vi "Add Step to Tree.vi"(9 "Step Index":i32, 10 "Step Settings":T1, 11 "UI Data In":refnum<class "Settings UI.lvclass">) -> (1 "Tree Items":T2(array[cluster]), 2 "Step tag":string, 3 "UI Data out":refnum<class "Settings UI.lvclass">)   [LabVIEW 2020, in "Output Sequencer.lvlib" / "Settings UI.lvclass"]
uses:
  Settings UI.lvclass
  Types/Step Settings.ctl
  Types/Tree Index Enum.ctl
  Globals/Global Tree Data.vi
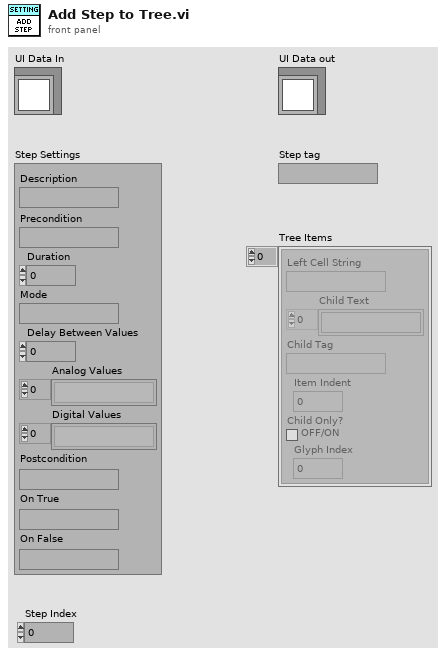
[diagram p1: front panel]
types:
  T1 = typedef "Output Sequencer.lvlib/Settings UI.lvclass/Step Settings.ctl" = cluster{"Description":string, "Precondition":string, "Duration":dbl, "Mode":string, "Delay Between Values":dbl, "Analog Values":string[], "Digital Values":string[], "Postcondition":string, "On True":string, "On False":string}
  T2 = cluster{"Left Cell String":string, "Child Text":string[], "Child Tag":string, "Item Indent":i32, "Child Only?":bool, "Glyph Index":i32}[]
  T3 = typedef "Output Sequencer.lvlib/Settings UI.lvclass/Tree Index Enum.ctl" = enum16{"General Settings", "Num Steps", "Num Analog", "Num Digital", "Show Confirmation", "Interp Priority", "Adv Timing", "Enable Conditions", "Seq Execution", "Reset Test Start", "Only When Test", "Delay After Test", "Start condition", "Re-triggering", "Stop condition", "Stop After Cycles", "Stop Values", "Default Values", "Default Analog", "Default Digital", "Steps", "Step #", "Description", "Precondition", "Duration", "Mode", "Delay Between Vals", "Analog Values", "Digital Values", "Postcondition", "On True", "On False"}
  T4 = cluster{"Left Cell String":string, "Child Text":string[], "Child Tag":string, "Item Indent":i32, "Child Only?":bool, "Glyph Index":i32}
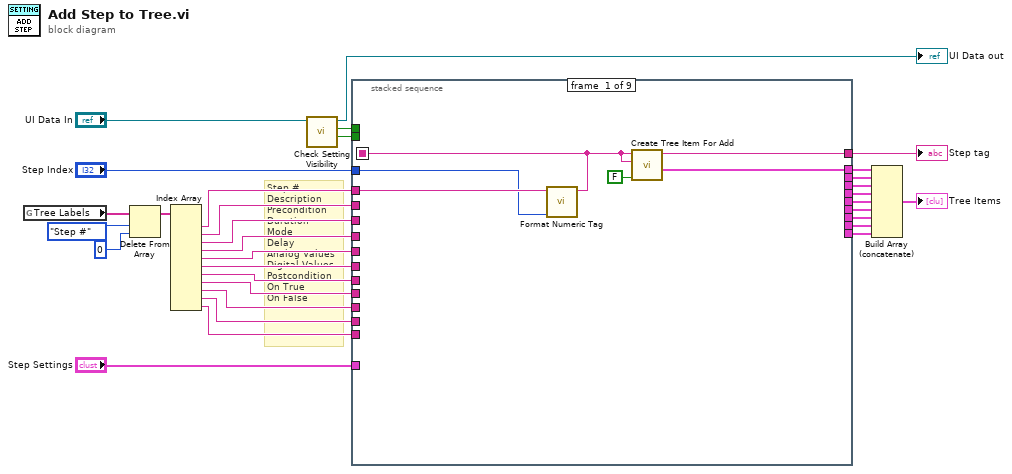
[diagram p0: block diagram]
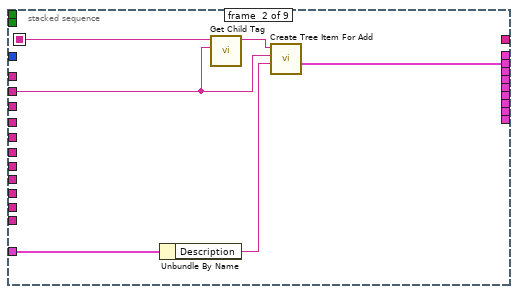
[diagram p2: hidden frame]
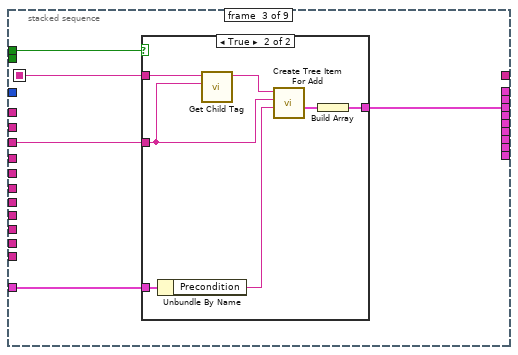
[diagram p3: hidden frame]
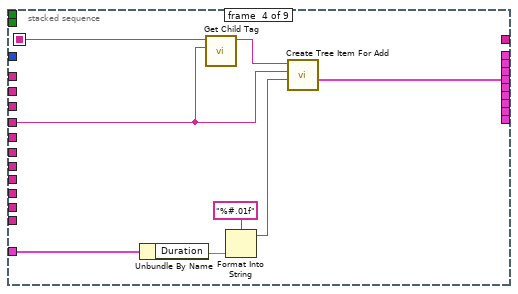
[diagram p5: hidden frame]
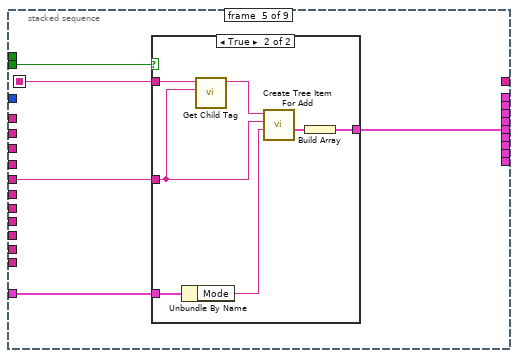
[diagram p6: hidden frame]
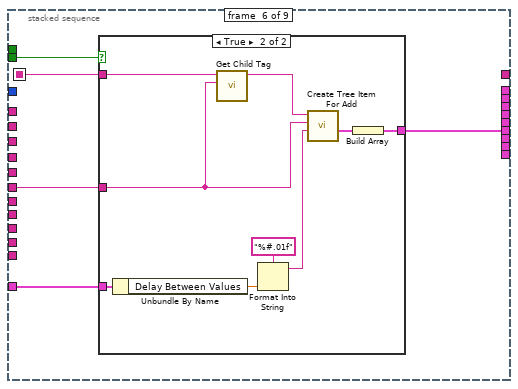
[diagram p8: hidden frame]
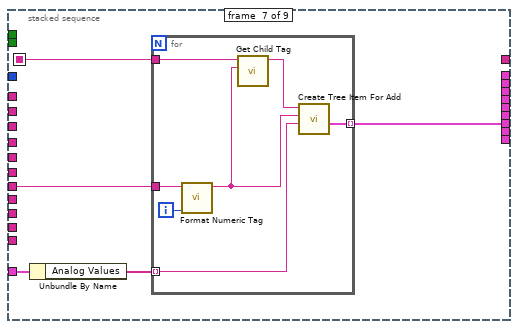
[diagram p10: hidden frame]
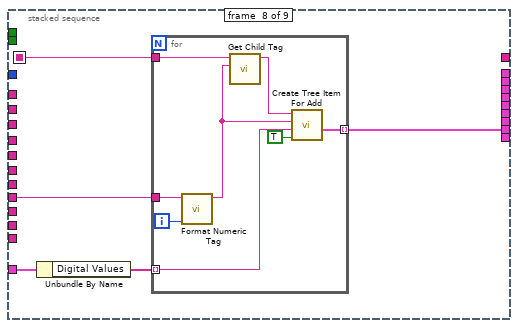
[diagram p11: hidden frame]
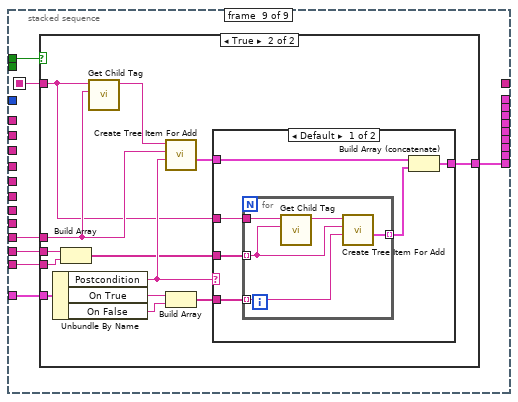
[diagram p12: hidden frame]
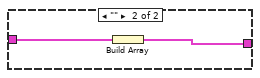
[diagram p14: hidden frame]
diagram:
  # "Step #\nDescription\nPrecondition\nDuration\nMode\nDelay\nAnalog Values\nDigital Values\nPostcondition\nOn True\nOn False"
  n1 = global read "Global Tree Data.vi" "Tree Labels"() -> (w14:string[])
  n2 = Delete From Array(array=w14, length=Tree_Index_Enum."Step #" ("Tree Index Enum"), index=0) -> (array with subset deleted=w21:string[])  [unwired: 1 out]
  n3 = Index Array(array=w21) -> (element #1=w20:string, element #2=w16:string, element #3=w17:string, element #4=w18:string, element #5=w19:string, element #6=w15:string, element #7=w13:string, element #8=w11:string, element #9=w9:string, element #10=w8:string, element #11=w7:string)  [unwired: 11 in]
  n4 = call "Check Setting Visibility.vi"("UI Data in"="UI Data In") -> ("Advanced timing visible"=w3:bool, "Conditional settings visible"=w2:bool, "UI Data out"=→"UI Data out":refnum<class "Settings UI.lvclass">)  [unwired: 7 in, 1 out]
  n5 = stacked-sequence {
    seq-local: [w33 _ _ _ _ _ _ _ _] -> [_ w41 w49 w59 w69 w81 w95 w107 w119]
    tunnel: "Step Index" -> [w34 _ _ _ _ _ _ _ _]
    tunnel: w20 -> [w35 _ _ _ _ _ _ _ _]
    tunnel: [w37 _ _ _ _ _ _ _ _] -> w29
    tunnel: w16 -> [_ w40 _ _ _ _ _ _ _]
    tunnel: [w38 _ _ _ _ _ _ _ _] -> w23
    tunnel: [_ _ w47 _ _ _ _ _ _] -> w24
    tunnel: "Step Settings" -> [_ w44 w48 w64 w68 w80 w92 w104 w122]
    tunnel: w17 -> [_ _ w46 _ _ _ _ _ _]
    tunnel: [_ _ _ w60 _ _ _ _ _] -> w25
    tunnel: w18 -> [_ _ _ w58 _ _ _ _ _]
    tunnel: w3 -> [_ _ _ _ w67 w79 _ _ _]
    tunnel: [_ _ _ _ w65 _ _ _ _] -> w26
    tunnel: w19 -> [_ _ _ _ w66 _ _ _ _]
    tunnel: [_ _ _ _ _ w77 _ _ _] -> w27
    tunnel: [_ _ _ _ _ _ w93 _ _] -> w28
    tunnel: w15 -> [_ _ _ _ _ w78 _ _ _]
    tunnel: w13 -> [_ _ _ _ _ _ w94 _ _]
    tunnel: [_ w43 _ _ _ _ _ _ _] -> w12
    tunnel: w11 -> [_ _ _ _ _ _ _ w106 _]
    tunnel: [_ _ _ _ _ _ _ w105 _] -> w10
    tunnel: w9 -> [_ _ _ _ _ _ _ _ w121]
    tunnel: w8 -> [_ _ _ _ _ _ _ _ w118]
    tunnel: w7 -> [_ _ _ _ _ _ _ _ w117]
    tunnel: [_ _ _ _ _ _ _ _ w120] -> w6
    tunnel: w2 -> [_ _ w45 _ _ _ _ _ w116]
    frame #0 {
      n6 = call "Format Numeric Tag.vi"("Number"=w34, "Tree label"=w35) -> ("Tag"=w33:string)  [unwired: 9 in]
      n7 = call "Create Tree Item For Add.vi"("Child Only? (true)"=FALSE ("Child Only?"), "Left Cell String"=w33, "Child Tag in"=w33) -> ("Item"=w38:T4, "Child Tag out"=w37:string)  [unwired: 7 in]
    }
    frame #1 {
      n8 = Unbundle By Name(w44) -> ("Description"=w42:string)
      n9 = call "Get Child Tag.vi"("Child label"=w40, "Parent tag"=w41) -> ("Child tag"=w39:string)  [unwired: 9 in]
      n10 = call "Create Tree Item For Add.vi"("Child Text"=w42, "Left Cell String"=w40, "Child Tag in"=w39) -> ("Item"=w43:T4)  [unwired: 7 in, 1 out]
    }
    frame #2 {
      n11 = case shown="True" w45 {
        tunnel: w49 -> [_ w52]
        tunnel: w48 -> [_ w56]
        tunnel: [_ w54] -> w47
        tunnel: w46 -> [_ w51]
        frame False {
        }
        frame True {
          n12 = Unbundle By Name(w56) -> ("Precondition"=w55:string)
          n13 = call "Get Child Tag.vi"("Child label"=w51, "Parent tag"=w52) -> ("Child tag"=w50:string)  [unwired: 9 in]
          n14 = call "Create Tree Item For Add.vi"("Child Text"=w55, "Left Cell String"=w51, "Child Tag in"=w50) -> ("Item"=w53:T4)  [unwired: 7 in, 1 out]
          n15 = Build Array(w53) -> (w54:T2)
        }
      }
    }
    frame #3 {
      n16 = Unbundle By Name(w64) -> ("Duration"=w63:dbl)
      n17 = call "Get Child Tag.vi"("Child label"=w58, "Parent tag"=w59) -> ("Child tag"=w57:string)  [unwired: 9 in]
      n18 = Format Into String(format string="%#.01f", w63) -> (resulting string=w61:string)  [unwired: 2 in, 1 out]
      n19 = call "Create Tree Item For Add.vi"("Child Text"=w61, "Left Cell String"=w58, "Child Tag in"=w57) -> ("Item"=w60:T4)  [unwired: 7 in, 1 out]
    }
    frame #4 {
      n20 = case shown="True" w67 {
        tunnel: w69 -> [_ w71]
        tunnel: w68 -> [_ w76]
        tunnel: w66 -> [_ w72]
        tunnel: [_ w74] -> w65
        frame False {
        }
        frame True {
          n21 = Unbundle By Name(w76) -> ("Mode"=w73:string)
          n22 = call "Get Child Tag.vi"("Child label"=w72, "Parent tag"=w71) -> ("Child tag"=w70:string)  [unwired: 9 in]
          n23 = call "Create Tree Item For Add.vi"("Child Text"=w73, "Left Cell String"=w72, "Child Tag in"=w70) -> ("Item"=w75:T4)  [unwired: 7 in, 1 out]
          n24 = Build Array(w75) -> (w74:T2)
        }
      }
    }
    frame #5 {
      n25 = case shown="True" w79 {
        tunnel: w81 -> [_ w83]
        tunnel: w80 -> [_ w90]
        tunnel: [_ w88] -> w77
        tunnel: w78 -> [_ w84]
        frame False {
          # "If no analog or digital channels configured, no need for delay since this only applies to channels."
        }
        frame True {
          n26 = Unbundle By Name(w90) -> ("Delay Between Values"=w86:dbl)
          n27 = call "Get Child Tag.vi"("Child label"=w84, "Parent tag"=w83) -> ("Child tag"=w82:string)  [unwired: 9 in]
          n28 = Format Into String(format string="%#.01f", w86) -> (resulting string=w85:string)  [unwired: 2 in, 1 out]
          n29 = call "Create Tree Item For Add.vi"("Child Text"=w85, "Left Cell String"=w84, "Child Tag in"=w82) -> ("Item"=w89:T4)  [unwired: 7 in, 1 out]
          n30 = Build Array(w89) -> (w88:T2)
        }
      }
    }
    frame #6 {
      n31 = Unbundle By Name(w92) -> ("Analog Values"=w91:string[])
      n32 = for {
        tunnel: w95 -> [w100]
        tunnel: w94 -> [w98]
        tunnel: [w102] -> w93 mode=indexing
        tunnel: w91 -> [w101] mode=indexing
        i -> [w97]
        n33 = call "Format Numeric Tag.vi"("Number"=w97, "Tree label"=w98) -> ("Tag"=w96:string)  [unwired: 9 in]
        n34 = call "Get Child Tag.vi"("Child label"=w96, "Parent tag"=w100) -> ("Child tag"=w99:string)  [unwired: 9 in]
        n35 = call "Create Tree Item For Add.vi"("Child Text"=w101, "Left Cell String"=w96, "Child Tag in"=w99) -> ("Item"=w102:T4)  [unwired: 7 in, 1 out]
      }
    }
    frame #7 {
      n36 = Unbundle By Name(w104) -> ("Digital Values"=w103:string[])
      n37 = for {
        tunnel: w107 -> [w112]
        tunnel: w106 -> [w110]
        tunnel: [w115] -> w105 mode=indexing
        tunnel: w103 -> [w114] mode=indexing
        i -> [w109]
        n38 = call "Format Numeric Tag.vi"("Number"=w109, "Tree label"=w110) -> ("Tag"=w108:string)  [unwired: 9 in]
        n39 = call "Get Child Tag.vi"("Child label"=w108, "Parent tag"=w112) -> ("Child tag"=w111:string)  [unwired: 9 in]
        n40 = call "Create Tree Item For Add.vi"("Child Only? (true)"=TRUE ("Child Only?"), "Child Text"=w114, "Left Cell String"=w108, "Child Tag in"=w111) -> ("Item"=w115:T4)  [unwired: 6 in, 1 out]
      }
    }
    frame #8 {
      n41 = case shown="True" w116 {
        tunnel: w122 -> [_ w135]
        tunnel: w121 -> [_ w125]
        tunnel: [_ w132] -> w120
        tunnel: w119 -> [_ w124]
        tunnel: w118 -> [_ w131]
        tunnel: w117 -> [_ w130]
        frame False {
        }
        frame True {
          n42 = Unbundle By Name(w135) -> ("Postcondition"=w134:string, "On True"=w129:string, "On False"=w128:string)
          n43 = Build Array(w131, w130) -> (w126:string[])
          n44 = call "Get Child Tag.vi"("Child label"=w125, "Parent tag"=w124) -> ("Child tag"=w123:string)  [unwired: 9 in]
          n45 = call "Create Tree Item For Add.vi"("Child Text"=w134, "Left Cell String"=w125, "Child Tag in"=w123) -> ("Item"=w133:T4)  [unwired: 7 in, 1 out]
          n46 = Build Array(w129, w128) -> (w127:string[])
          n47 = case shown="Default" w134 {
            tunnel: w133 -> [w138 w148]
            tunnel: [w137 w147] -> w132
            tunnel: w124 -> [w141 _]
            tunnel: w127 -> [w140 _]
            tunnel: w126 -> [w139 _]
            frame Default {
              n48 = for {
                tunnel: w141 -> [w144]
                tunnel: w140 -> [w146] mode=indexing
                tunnel: w139 -> [w143] mode=indexing
                tunnel: [w145] -> w136 mode=indexing
                n49 = call "Get Child Tag.vi"("Child label"=w143, "Parent tag"=w144) -> ("Child tag"=w142:string)  [unwired: 9 in]
                n50 = call "Create Tree Item For Add.vi"("Child Text"=w146, "Left Cell String"=w143, "Child Tag in"=w142) -> ("Item"=w145:T4)  [unwired: 7 in, 1 out]
              }
              n51 = Build Array (concatenate)(w138, w136) -> (w137:T2)
            }
            frame "" {
              n52 = Build Array(w148) -> (w147:T2)
            }
          }
        }
      }
    }
  }
  "Step tag" <- w29
  n53 = Build Array (concatenate)(w23, w12, w24, w25, w26, w27, w28, w10, w6) -> (→"Tree Items":T2)
